vi "Analyze Target.vi"(8 "Goal Width":dbl, 9 "Center Right":dbl, 10 "Center Left":dbl, 11 "Relevant Data":T1[](array[typedef])) -> (3 "What to do":string)   [LabVIEW 2015]
uses:
  References/Relevant Data.ctl
panel:
  in  "Goal Area":dbl
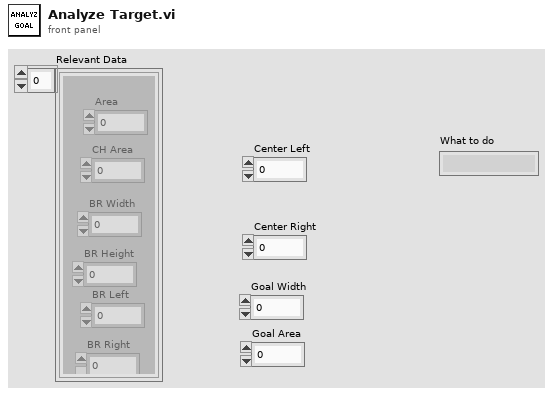
[diagram p1: front panel]
types:
  T1 = typedef "Relevant Data.ctl" = cluster{"Area":dbl, "CH Area":dbl, "BR Width":dbl, "BR Height":dbl, "BR Left":dbl, "BR Right":dbl}
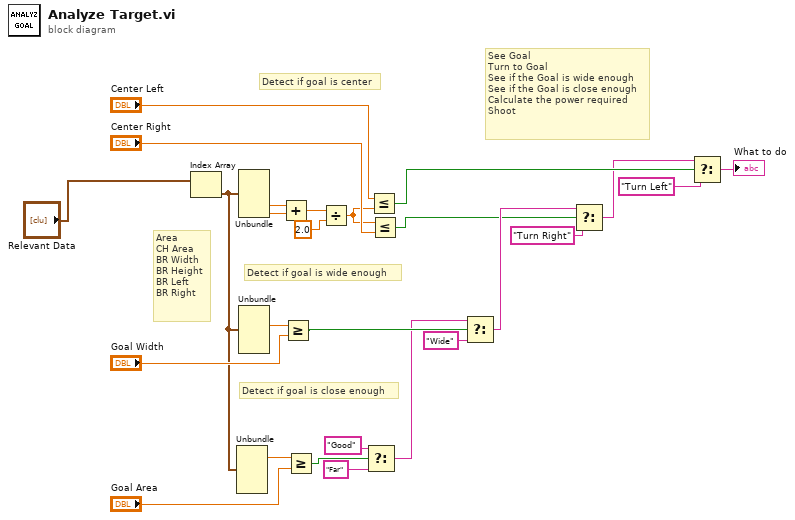
[diagram p0: block diagram]
diagram:
  # "See Goal\nTurn to Goal\nSee if the Goal is wide enough\nSee if the Goal is close enough\nCalculate the power required\nShoot"
  # "Detect if goal is close enough"
  # "Detect if goal is wide enough"
  # "Detect if goal is center"
  # "Area\nCH Area\nBR Width\nBR Height\nBR Left\nBR Right"
  n1 = Index Array(array="Relevant Data") -> (element=w16:T1)  [unwired: 1 in]
  n2 = Unbundle(w16) -> ("CH Area"=w15:dbl)  [unwired: 5 out]
  n3 = Unbundle(w16) -> ("BR Left"=w22:dbl, "BR Right"=w21:dbl)  [unwired: 4 out]
  n4 = Unbundle(w16) -> ("BR Width"=w17:dbl)  [unwired: 5 out]
  n5 = Add(x=w22, y=w21) -> (x+y=w20:dbl)
  n6 = Greater Or Equal?(x=w17, y="Goal Width") -> (x >= y?=w10:bool)
  n7 = Greater Or Equal?(x=w15, y="Goal Area") -> (x >= y?=w14:bool)
  n8 = Divide(x=w20, y=2.0) -> (x/y=w18:dbl)
  n9 = Select(t="Good", s=w14, f="Far") -> (s? t:f=w9:string)
  n10 = Less Or Equal?(x="Center Left", y=w18) -> (x <= y?=w4:bool)
  n11 = Less Or Equal?(x=w18, y="Center Right") -> (x <= y?=w5:bool)
  n12 = Select(t=w9, s=w10, f="Wide") -> (s? t:f=w7:string)
  n13 = Select(t=w7, s=w5, f="Turn Right") -> (s? t:f=w3:string)
  n14 = Select(t=w3, s=w4, f="Turn Left") -> (s? t:f=→"What to do":string)
